vi "setUp.vi"(8 "error in (no error)":errorcluster, 11 "reference in":refnum<class "System Monitor System Tests.lvclass">) -> (0 "error out":errorcluster, 3 "reference out":refnum<class "System Monitor System Tests.lvclass">)   [LabVIEW 2027, in "System Monitor System Tests.lvclass"]
doc: "setUp runs prior to the test method during test execution. Use this method to initialize any object data required by your tests."
uses:
  System Monitor System Tests.lvclass
  C:/Program Files/National Instruments/LabVIEW 2027/vi.lib/addons/_JKI Toolkits/VI Tester/TestCase.llb/TestCase.lvclass
  <vilib>/addons/_JKI Toolkits/VI Tester/TestCase.llb/TestCase.lvclass
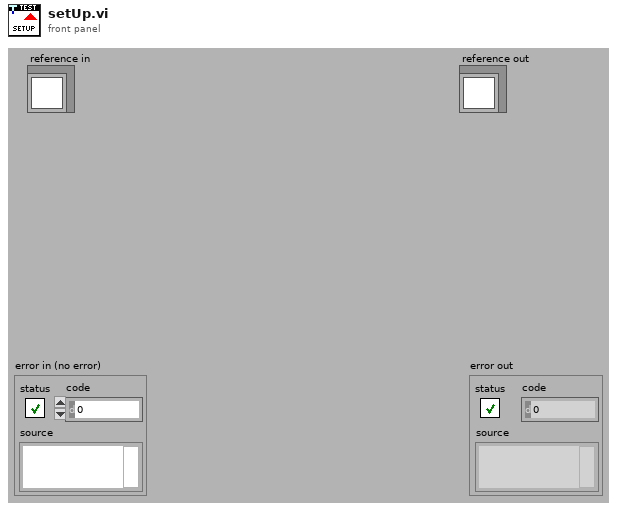
[diagram p1: front panel]
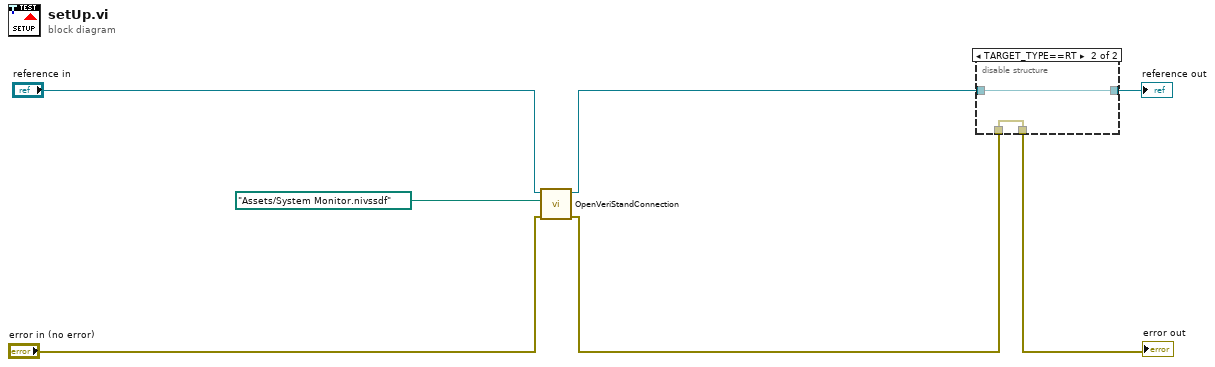
[diagram p0: block diagram]
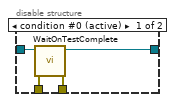
[diagram p2: hidden frame]
diagram:
  n1 = call-dynamic "OpenVeriStandConnection.vi"("error in (no error)"="error in (no error)", "System Definition File"=path "Assets/System Monitor.nivssdf", "VeriStand Test Case in"="reference in") -> ("error out"=w4:errorcluster, "VeriStand Test Case out"=w2:refnum<class "System Monitor System Tests.lvclass">)  [unwired: 6 in, 1 out]
  n2 = disable-structure shown="TARGET_TYPE==RT" {
    disable-tunnel: w4 -> [w11 w12]
    disable-tunnel: [w10 w12] -> w7
    disable-tunnel: [w9 w13] -> w6
    disable-tunnel: w2 -> [w8 w13]
    frame condition #0 (active) {
      n3 = call <vilib>:"WaitOnTestComplete.vi"("error in (no error)"=w11, "TestCase in"=w8) -> ("error out"=w10:errorcluster, "TestCase out"=w9:refnum<class "System Monitor System Tests.lvclass">)  [unwired: 8 in]
    }
    frame condition #1 {
    }
  }
  "error out" <- w7
  "reference out" <- w6
